vi "Populate Attributes Table.vi"(8 "error in":errorcluster, 10 "Index":string, 11 "UI Actor in":refnum<class "UI Actor.lvclass">) -> (0 "error out":errorcluster, 3 "UI Actor out":refnum<class "UI Actor.lvclass">)   [LabVIEW 2024, in "UI Actor.lvlib" / "UI Actor.lvclass"]
uses:
  UI Actor.lvclass
  UI Actor.lvclass/UI Actor.ctl
  Electronic Datasheet/Electronic Datasheet.lvclass
  Core/OD Entry/OD Entry.lvclass
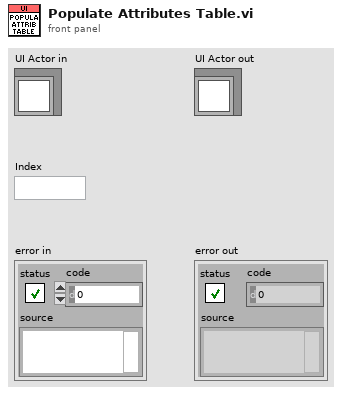
[diagram p1: front panel]
types:
  T1 = map{path, refnum<class "Electronic Datasheet.lvclass">}
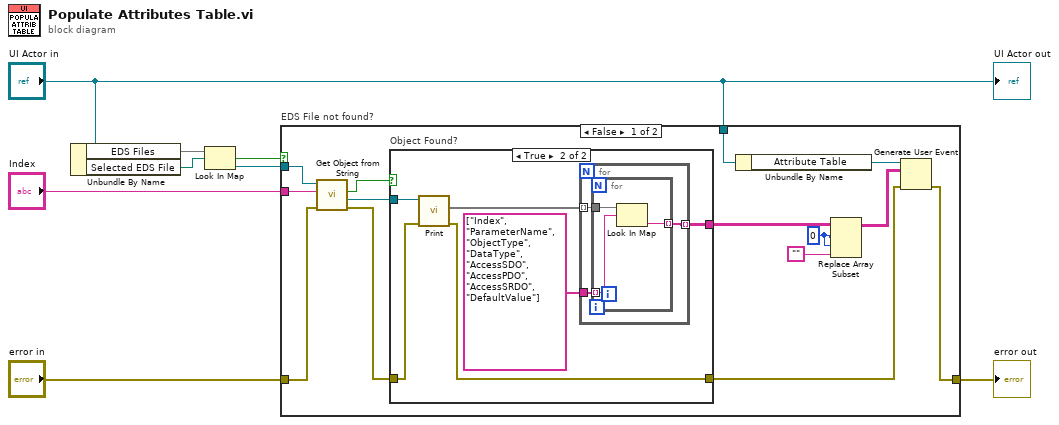
[diagram p0: block diagram]
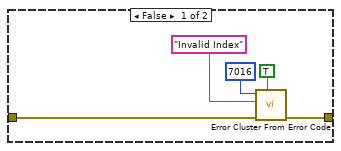
[diagram p2: hidden frame]
diagram:
  n1 = Unbundle By Name("UI Actor in") -> ("EDS Files"=w8:T1, "Selected EDS File"=w7:path)
  n2 = Look In Map(map=w8, key=w7) -> (key not found?=w2:bool, value=w6:refnum<class "Electronic Datasheet.lvclass">)  [unwired: 1 in]
  n3 = case "EDS File not found?" shown="False" w2 {
    tunnel: w6 -> [w11 _]
    tunnel: "error in" -> [w13 w40]
    tunnel: [w20 w40] -> w4
    tunnel: "UI Actor in" -> [w21 _]
    tunnel: "Index" -> [w14 _]
    frame False {
      w15 = 0 ("index (row)")
      n4 = call "Get Object from String.vi"("error in"=w13, "Index"=w14, "reference in"=w11) -> ("error out"=w12:errorcluster, "OD Entry"=w9:refnum<class "OD Entry.lvclass">, "Found?"=w10:bool)  [unwired: 5 in, 1 out]
      n5 = case "Object Found?" shown="True" w10 {
        tunnel: w12 -> [w27 w32]
        tunnel: [w26 w31] -> w19
        tunnel: w9 -> [_ w33]
        tunnel: [_ w28] -> w18
        frame False {
          n6 = call <vilib>:"Error Cluster From Error Code.vi"("show call chain? (False)"=TRUE, "error in (no error)"=w27, "error message (\"\")"="Invalid Index" ("error message (\"\")"), "error code (0)"=7016) -> ("error out"=w26:errorcluster)  [unwired: 5 in]
        }
        frame True {
          n7 = call "Print.vi"("error in"=w32, "OD Entry in"=w33) -> ("error out"=w31:errorcluster, "Entry with Sub-Entries"=w30:map{string, string}[])  [unwired: 7 in, 1 out]
          n8 = for {
            tunnel: w30 -> [w36] mode=indexing
            tunnel: string[] ["Index", "ParameterName", "ObjectType", "DataType", "AccessSDO", "AccessPDO", "AccessSRDO", "DefaultValue"] ("Compulsory Objects") -> [w35]
            tunnel: [w34] -> w28 mode=indexing
            n9 = for {
              tunnel: w36 -> [w39]
              tunnel: w35 -> [w38] mode=indexing
              tunnel: [w37] -> w34 mode=indexing
              n10 = Look In Map(map=w39, key=w38) -> (value=w37:string)  [unwired: 1 in, 1 out]
            }
          }
        }
      }
      n11 = Unbundle By Name(w21) -> ("Attribute Table"=w22:refnum<user-event>)
      n12 = Replace Array Subset(array=w18, new element="", index (row)=w15, index (col)=w15) -> (w17:string[][])
      n13 = Generate User Event(user event=w22, event data cluster=w17, error in=w19) -> (error out=w20:errorcluster)  [unwired: 1 in, 1 out]
    }
    frame True {
    }
  }
  "error out" <- w4
  "UI Actor out" <- "UI Actor in"
